vi "Configure Acquire.vi"(6 "Acquisition Mode (0: Normal)":i32(ring) items=["Normal", "Average", "Peak", "High Resolution"], 8 "error in (no error)":errorcluster, 9 "Waveform Point Number (0: Auto)":i32(ring) items=["Auto", "14000", "140000", "1400000", "14000000", "56000000", "112000000", "3500", "7000", "70000", "700000", "7000000", "28000000"], 10 "Average Number (2)":dbl=2.0, 11 "VISA resource name":refnum<visa-resource-name>) -> (0 "error out":errorcluster, 3 "VISA resource name out":refnum<visa-resource-name>)   [LabVIEW 2015, in "ZhiYuan ZDS Series for TCP.lvlib"]
doc: "Configures the setting for acquire system."
uses:
  ZhiYuan ZDS Series for TCP.lvlib
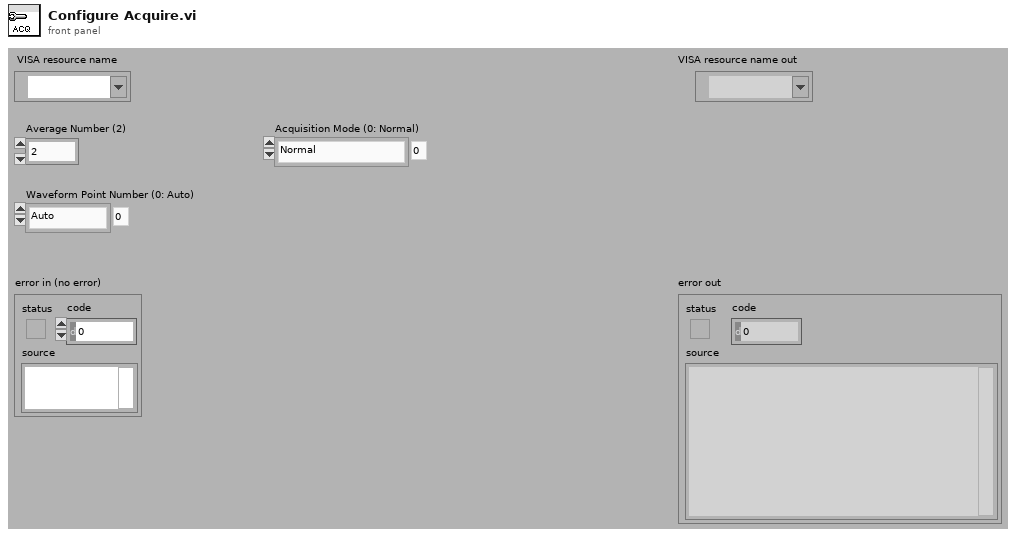
[diagram p1: front panel]
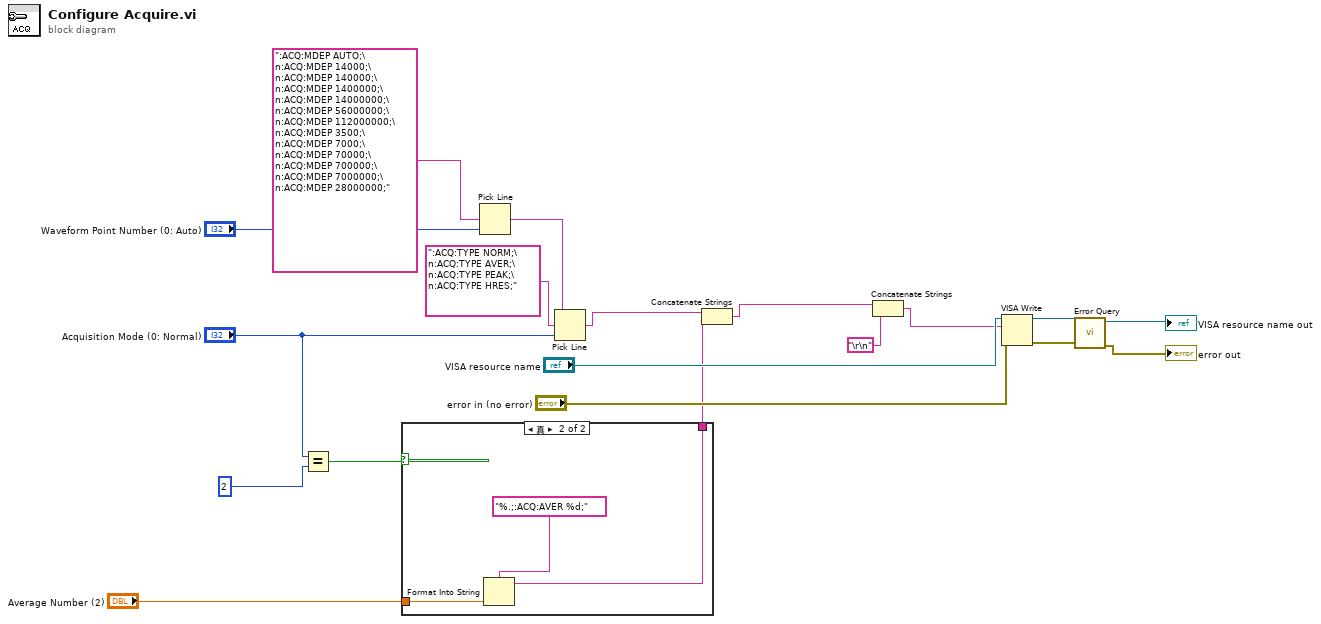
[diagram p0: block diagram]
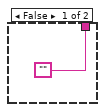
[diagram p2: hidden frame]
diagram:
  n1 = Equal?(x="Acquisition Mode (0: Normal)", y=2) -> (x = y?=w6:bool)
  n2 = case shown="真" w6 {
    tunnel: "Average Number (2)" -> [_ w22]
    tunnel: ["" w21] -> w1
    frame False {
    }
    frame True {
      n3 = Format Into String(format string="%.;:ACQ:AVER %d;", w22) -> (resulting string=w21:string)  [unwired: 2 in, 1 out]
    }
  }
  n4 = Pick Line(multi-line string=":ACQ:MDEP AUTO;\n:ACQ:MDEP 14000;\n:ACQ:MDEP 140000;\n:ACQ:MDEP 1400000;\n:ACQ:MDEP 14000000;\n:ACQ:MDEP 56000000;\n:ACQ:MDEP 112000000;\n:ACQ:MDEP 3500;\n:ACQ:MDEP 7000;\n:ACQ:MDEP 70000;\n:ACQ:MDEP 700000;\n:ACQ:MDEP 7000000;\n:ACQ:MDEP 28000000;", line index="Waveform Point Number (0: Auto)") -> (output string=w16:string)  [unwired: 1 in]
  n5 = Pick Line(string ("")=w16, multi-line string=":ACQ:TYPE NORM;\n:ACQ:TYPE AVER;\n:ACQ:TYPE PEAK;\n:ACQ:TYPE HRES;", line index="Acquisition Mode (0: Normal)") -> (output string=w3:string)
  n6 = Concatenate Strings(w3, w1) -> (w2:string)
  n7 = Concatenate Strings(w2, "\r\n") -> (w8:string)
  n8 = VISA Write(VISA resource name="VISA resource name", write buffer=w8, error in (no error)="error in (no error)") -> (VISA resource name out=w12:refnum<visa-resource-name>, error out=w13:errorcluster)  [unwired: 1 out]
  n9 = call "Error Query.vi"("error in (no error)"=w13, "VISA resource name"=w12) -> ("error out"=→"error out":errorcluster, "VISA resource name out"=→"VISA resource name out":refnum<visa-resource-name>)  [unwired: 6 in, 2 out]
